vi "set_model_doc.vi"(8 "error in":errorcluster, 10 "Array":string[](array[string])=["tree", "DecisionTreeClassifier", "fit"], 11 "vi refnum":refnum<vi>) -> (0 "error out":errorcluster, 3 "reference out":refnum<vi>)   [LabVIEW 2020]
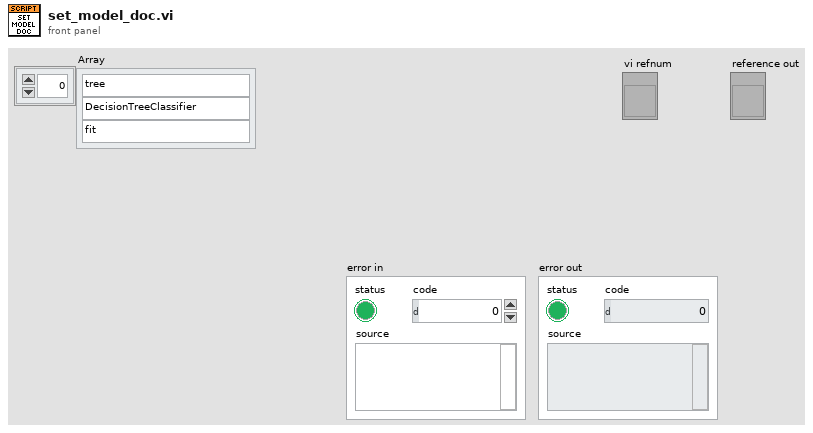
[diagram p1: front panel]
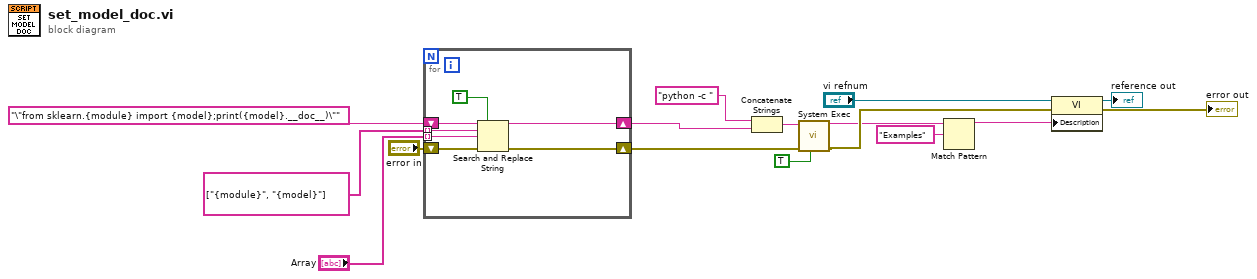
[diagram p0: block diagram]
diagram:
  n1 = for {
    tunnel: string[] ["{module}", "{model}"] -> [w22] mode=indexing
    shift-right: [w20] -> w10
    shift-left: "\"from sklearn.{module} import {model};print({model}.__doc__)\"" ("standard input") -> [w23]
    tunnel: "Array" -> [w21] mode=indexing
    shift-right: [w19] -> w13
    shift-left: "error in" -> [w18]
    n2 = Search and Replace String(replace all?=TRUE ("replace all? (F)"), input string=w23, search string=w22, replace string=w21, error in=w18) -> (result string=w20:string, error out=w19:errorcluster)  [unwired: 3 in, 2 out]
  }
  n3 = Concatenate Strings("python -c " ("command line"), w10) -> (w12:string)
  n4 = call <vilib>:"System Exec.vi"("run minimized? (F)"=TRUE, "error in (no error)"=w13, "command line"=w12) -> ("error out"=w4:errorcluster, "standard output"=w3:string)  [unwired: 5 in, 2 out]
  n5 = Match Pattern(string=w3, regular expression="Examples") -> (before substring=w2:string)  [unwired: 1 in, 3 out]
  n6 = property class="VI"(reference="vi refnum", error in=w4, "Description"=w2) -> (reference out=→"reference out":refnum<vi>, error out=→"error out":errorcluster)
